vi "ConnectAsGRPC.vi"(8 "error in":errorcluster, 11 "Connection String":string) -> (0 "error out":errorcluster, 3 "MicronClient out":refnum<class "MicronClient.lvclass">)   [LabVIEW 2019, in "MicronGRPCClient.lvclass"]
uses:
  MicronGRPCClient.lvclass
  Base/Client/MicronClient.lvclass
  D:/GitHub/KarthikAbiram/Micron/Source/Base/Client/MicronClient.lvclass
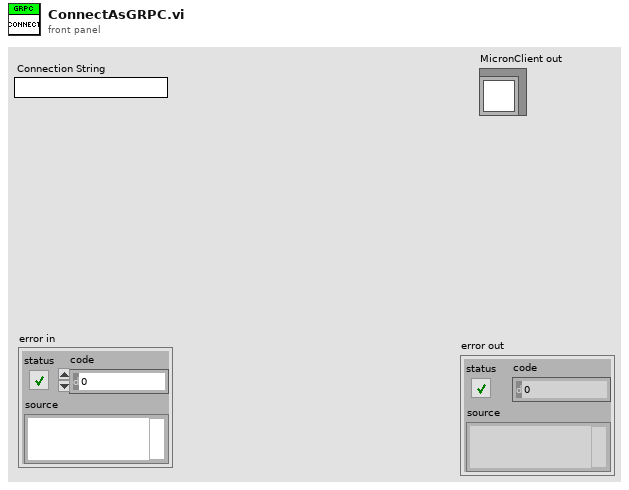
[diagram p1: front panel]
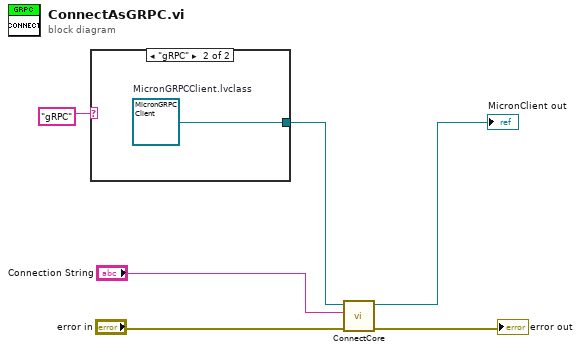
[diagram p0: block diagram]
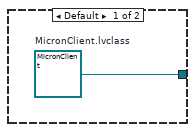
[diagram p2: hidden frame]
diagram:
  n1 = case shown="\"gRPC\"" "gRPC" {
    tunnel: [w7 w8] -> w4
    frame Default {
      w7 = refnum<class "MicronClient.lvclass"> refnum  # MicronClient.lvclass
    }
    frame "gRPC" {
      w8 = refnum<class "MicronGRPCClient.lvclass"> refnum  # MicronGRPCClient.lvclass
    }
  }
  n2 = call-dynamic "ConnectCore.vi"("error in (no error)"="error in", "Connection String"="Connection String", "MicronClient in"=w4) -> ("error out"=→"error out":errorcluster, "MicronClient out"=→"MicronClient out":refnum<class "MicronClient.lvclass">)  [unwired: 7 in]
